vi "VerifySignature (Public Key Bytes).vi"(5 "RSASignPadding":T2, 7 "HashingAlgorithm":T1=enum."SHA512", 8 "error in (no error)":errorcluster, 9 "Signature in":u8[](array[numeric]), 10 "Data in":u8[](array[numeric]), 11 "Public key in":u8[](array[numeric])) -> (0 "error out":errorcluster, 2 "Verified?":bool)   [LabVIEW 2021, in "dotNET Crypto Asymmetric Encryption.lvlib"]
doc: "Verify the signature of the data using the public key."
uses:
  dotNET Crypto Asymmetric Encryption.lvlib
  RSASignaturePadding.ctl
  HashingAlgorithm.ctl
  System.Core
  Utility/dotNET Crypto Utility.lvlib
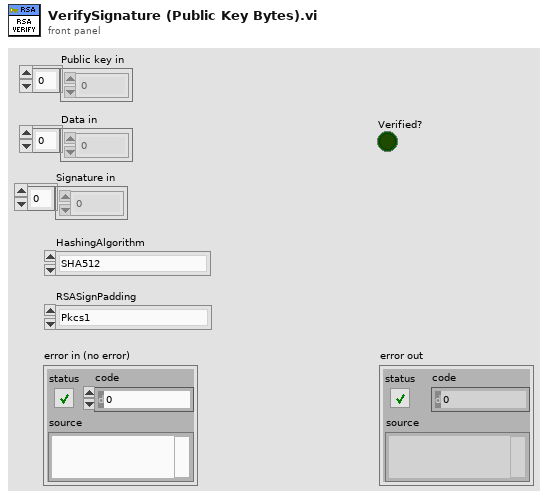
[diagram p1: front panel]
types:
  T1 = typedef "dotNET Crypto Utility.lvlib/HashingAlgorithm.ctl" = enum16{"MD5", "SHA1", "SHA256", "SHA384", "SHA512"}
  T2 = typedef "dotNET Crypto Asymmetric Encryption.lvlib/RSASignaturePadding.ctl" = enum16{"Pkcs1", "Pss"}
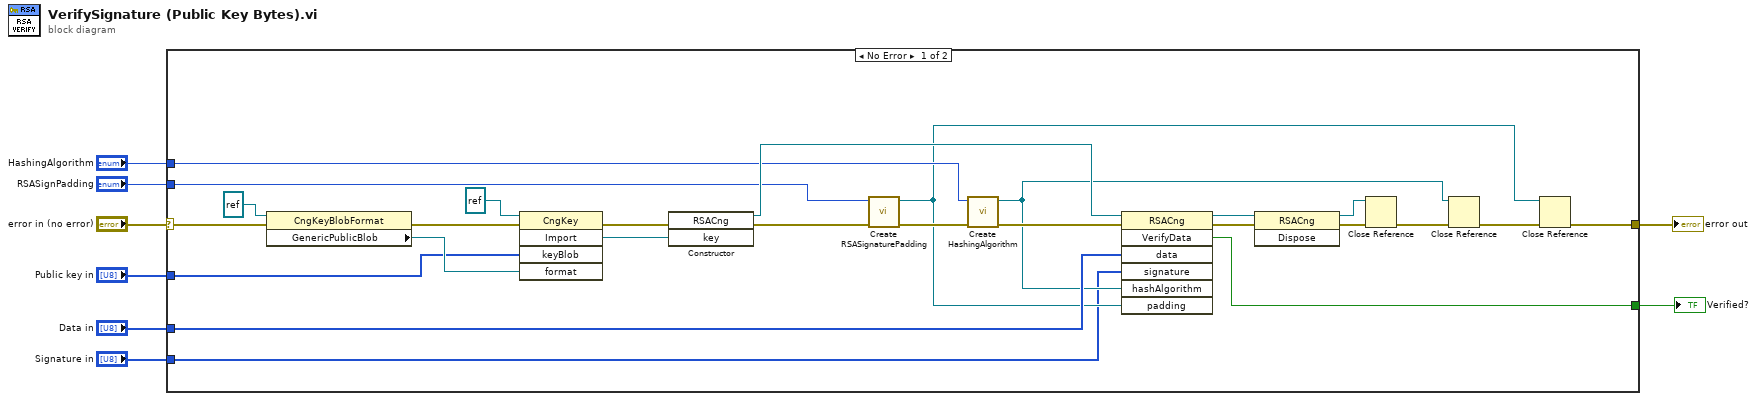
[diagram p0: block diagram]
diagram:
  n1 = case shown="No Error" "error in (no error)" {
    selector: "error in (no error)" -> [w12 w35]
    tunnel: "Data in" -> [w34 _]
    tunnel: "RSASignPadding" -> [w27 _]
    tunnel: "HashingAlgorithm" -> [w22 _]
    tunnel: [w19 _] -> w5
    tunnel: "Signature in" -> [w18 _]
    tunnel: [w17 w35] -> w3
    tunnel: "Public key in" -> [w9 _]
    frame No Error {
      n2 = property class="CngKeyBlobFormat"(reference=refnum<k24> refnum ("format"), error in=w12) -> (error out=w14:errorcluster, "GenericPublicBlob"=w13:refnum<k24>)  [unwired: 1 out]
      n3 = invoke class="CngKey" method="Import"(reference=refnum<k24> refnum, error in=w14, "keyBlob"=w9, "format"=w13) -> (error out=w11:errorcluster, "Import"=w10:refnum<k24>)  [unwired: 1 in, 3 out]
      n4 = constructor class="RSACng"(error in=w11, "key"=w10) -> (reference out=w28:refnum<k24>, error out=w29:errorcluster)  [unwired: 2 in, 2 out]
      n5 = call "Create RSASignaturePadding.vi"("error in (no error)"=w29, "RSASignaturePadding"=w27) -> ("error out"=w26:errorcluster, "RSASignaturePadding out"=w21:refnum<k24>)  [unwired: 8 in]
      n6 = call "Create HashingAlgorithm.vi"("error in (no error)"=w26, "HashingAlgorithm"=w22) -> ("error out"=w25:errorcluster, "Hashing Algorithm"=w20:refnum<k24>)  [unwired: 8 in]
      n7 = invoke class="RSACng" method="VerifyData"(reference=w28, error in=w25, "data"=w34, "signature"=w18, "hashAlgorithm"=w20, "padding"=w21) -> (reference out=w32:refnum<k24>, error out=w33:errorcluster, "VerifyData"=w19:bool)  [unwired: 1 in, 4 out]
      n8 = invoke class="RSACng" method="Dispose"(reference=w32, error in=w33) -> (reference out=w31:refnum<k24>, error out=w30:errorcluster)  [unwired: 1 in, 1 out]
      n9 = Close Reference(reference=w31, error in (no error)=w30) -> (error out=w24:errorcluster)
      n10 = Close Reference(reference=w20, error in (no error)=w24) -> (error out=w23:errorcluster)
      n11 = Close Reference(reference=w21, error in (no error)=w23) -> (error out=w17:errorcluster)
    }
    frame Error {
    }
  }
  "error out" <- w3
  "Verified?" <- w5
